vi "close.vi"(8 "error in":errorcluster, 11 "module in":refnum<class "DAQmx Watchdog runtime.lvclass">) -> (0 "error out":errorcluster)   [LabVIEW 2014, in "DAQmx Watchdog runtime.lvclass"]
doc: "Provides an interface for terminating a module instance. While this interface performs no operations, a child should close and deallocate any open references or memory."
uses:
  DAQmx Watchdog runtime.lvclass
  DAQmx Watchdog runtime.lvclass/DAQmx Watchdog runtime.ctl
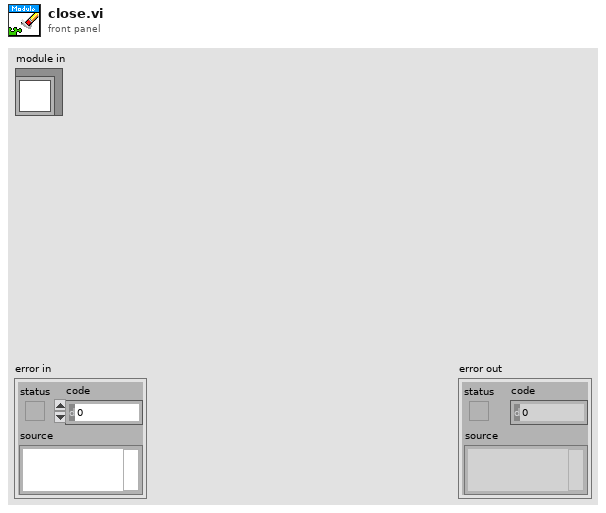
[diagram p1: front panel]
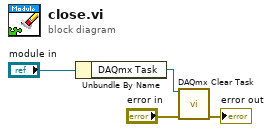
[diagram p0: block diagram]
diagram:
  n1 = Unbundle By Name("module in") -> ("DAQmx Task"=w2:refnum<k21>)
  n2 = call <vilib>:"DAQmx Clear Task.vi"("task in"=w2, "error in"="error in") -> ("error out"=→"error out":errorcluster)  [unwired: 13 in]
